vi "bt.vi"(6 "commants details":T1(array[cluster]), 7 "sending command":u8[](array[numeric]) format="%1d", 8 "connection in":refnum<k31>) -> (0 "check buffer error":errorcluster, 1 "reapons char error":errorcluster, 2 "received values":u8[](array[numeric]), 3 "income command id":u8, 4 "sending error":errorcluster, 5 "connection out":refnum<k31>)   [LabVIEW 2012]
panel:
  out "string sending command":string
  out "respons char":string
  out "income command id":string
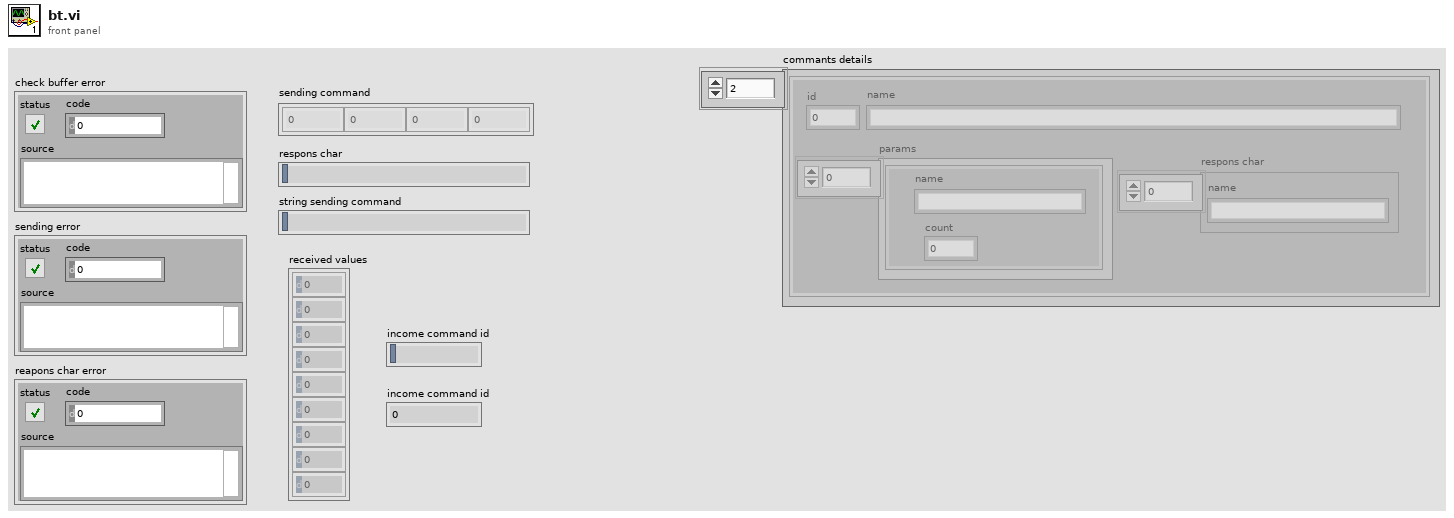
[diagram p1: front panel]
types:
  T1 = cluster{"id":u8, "name":string, "params":cluster{"name":string, "count":u8}[], "respons char":string[]}[]
  T2 = enum16{"Standard", "Buffered", "CRLF", "Immediate"}
  T3 = cluster{"id":u8, "name":string, "params":cluster{"name":string, "count":u8}[], "respons char":string[]}
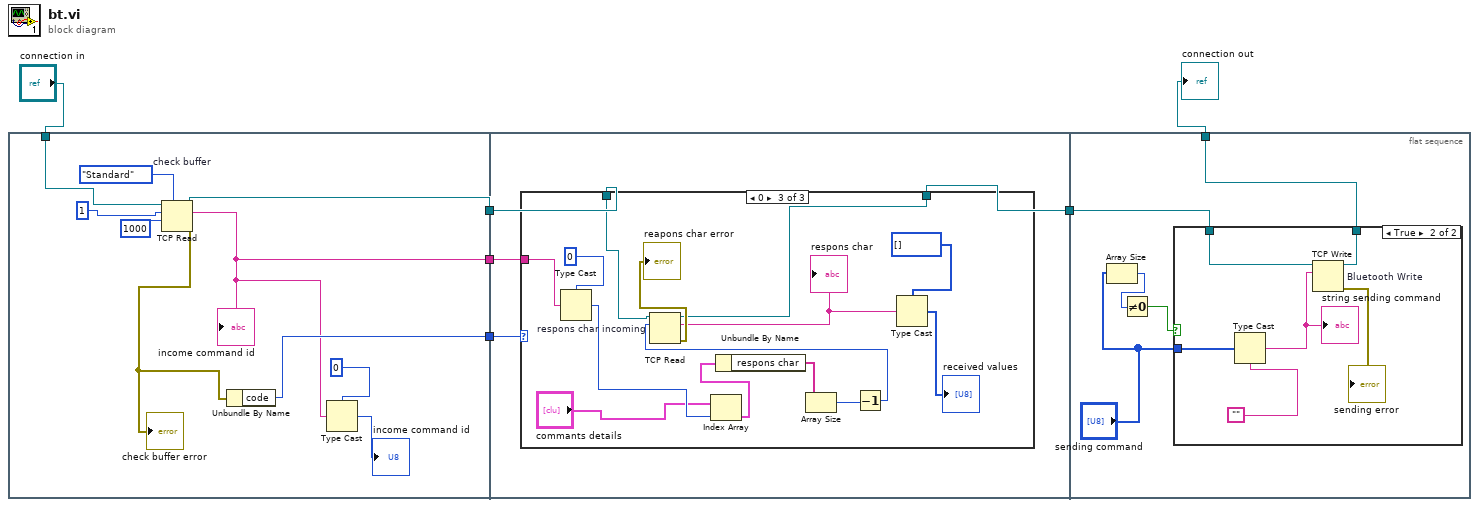
[diagram p0: block diagram]
diagram:
  n1 = flat-sequence {
    tunnel: "connection in" -> [w12]
    tunnel: [w16] -> w5
    tunnel: [w10] -> w4
    tunnel: [w8] -> w3
    tunnel: w5 -> [w18]
    tunnel: w4 -> [w20]
    tunnel: w3 -> [w19]
    tunnel: [w17] -> w2
    tunnel: [w37] -> w1
    tunnel: w2 -> [w41]
    frame #0 {
      n2 = TCP Read "check buffer"(connection ID=w12, bytes to read=1, 7:T2."Standard" ("mode (standard)"), 9:1000 ("timeout ms (25000)")) -> (connection ID out=w16:refnum<k31>, data out=w8:string, error out=w11:errorcluster)  [unwired: 1 in]
      "check buffer error" <- w11
      "income command id" <- w8
      n3 = Unbundle By Name(w11) -> ("code"=w10:i32)
      n4 = Type Cast(type=u8 0, x=w8) -> (*(type *) &x=→"income command id":u8)
    }
    frame #1 {
      n5 = case shown="0" w20 {
        tunnel: w19 -> [_ _ w36]
        tunnel: w18 -> [w21 w22 w34]
        tunnel: [w21 w22 w29] -> w17
        frame 56 {
        }
        frame Default {
        }
        frame 0 {
          n6 = Type Cast(type=u8 0, x=w36) -> (*(type *) &x=w33:u8)
          n7 = Index Array(array="commants details", index=w33) -> (element=w32:T3)
          n8 = Unbundle By Name(w32) -> ("respons char"=w31:string[])
          n9 = Array Size(array=w31) -> (size(s)=w24:i32)
          n10 = Decrement(x=w24) -> (x-1=w23:i32)
          n11 = TCP Read "respons char incoming"(connection ID=w34, bytes to read=w23) -> (connection ID out=w29:refnum<k31>, data out=w28:string, error out=→"reapons char error":errorcluster)  [unwired: 3 in]
          "respons char" <- w28
          n12 = Type Cast(type=u8[] [], x=w28) -> (*(type *) &x=→"received values":u8[])
        }
      }
    }
    frame #2 {
      n13 = Array Size(array="sending command") -> (size(s)=w39:i32)
      n14 = Not Equal To 0?(x=w39) -> (x != 0?=w38:bool)
      n15 = case shown="True" w38 {
        tunnel: "sending command" -> [_ w48]
        tunnel: w41 -> [w42 w46]
        tunnel: [w42 w45] -> w37
        frame False {
        }
        frame True {
          n16 = Type Cast(type="", x=w48) -> (*(type *) &x=w43:string)
          "string sending command" <- w43
          n17 = TCP Write "Bluetooth Write"(connection ID=w46, data in=w43) -> (connection ID out=w45:refnum<k31>, error out=→"sending error":errorcluster)  [unwired: 2 in, 1 out]
        }
      }
    }
  }
  "connection out" <- w1
